vi "Dispose ListView.vi"(8 "error in (no error)":errorcluster caption="错误输入（无错误）", 11 "ListViewClass 输入":refnum<class "ListViewClass.lvclass"> caption="DNL_LabVIEW Object in") -> (0 "error out":errorcluster caption="错误输出", 3 "ListViewClass 输出":refnum<class "ListViewClass.lvclass"> caption="DNL_LabVIEW Object out")   [LabVIEW 2012, in "ListViewClass.lvclass"]
uses:
  ListViewClass.lvclass
  ListViewClass.lvclass/ListViewClass.ctl
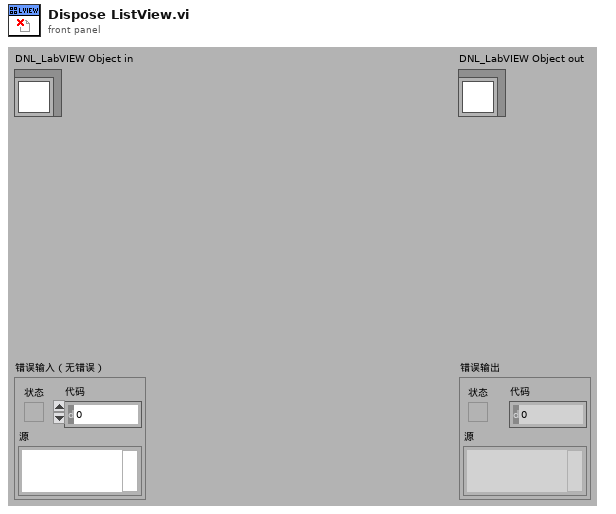
[diagram p1: front panel]
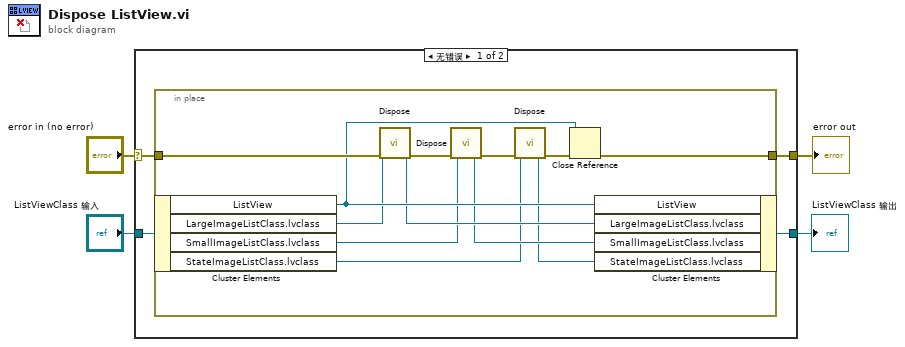
[diagram p0: block diagram]
diagram:
  n1 = case shown="无错误" "error in (no error)" {
    selector: "error in (no error)" -> [w8 w22]
    tunnel: [w7 w22] -> w3
    tunnel: [w5 w21] -> w1
    tunnel: "ListViewClass 输入" -> [w6 w21]
    frame No Error {
      n2 = in-place {
        in-place-border: w8 -> [w20]
        in-place-border: [w16] -> w7
        n3 = in-place-cluster #1(w6) -> ("ListView"=w15:refnum<k24>, "LargeImageListClass.lvclass"=w14:refnum<class "ImageListClass.lvclass">, "SmallImageListClass.lvclass"=w12:refnum<class "ImageListClass.lvclass">, "StateImageListClass.lvclass"=w10:refnum<class "ImageListClass.lvclass">)
        n4 = call "Dispose.vi"("error in (no error)"=w20, "ImageListClass 输入"=w14) -> ("error out"=w19:errorcluster, "ImageListClass 输出"=w13:refnum<class "ImageListClass.lvclass">)  [unwired: 8 in]
        n5 = call "Dispose.vi"("error in (no error)"=w19, "ImageListClass 输入"=w12) -> ("error out"=w18:errorcluster, "ImageListClass 输出"=w11:refnum<class "ImageListClass.lvclass">)  [unwired: 8 in]
        n6 = call "Dispose.vi"("error in (no error)"=w18, "ImageListClass 输入"=w10) -> ("error out"=w17:errorcluster, "ImageListClass 输出"=w9:refnum<class "ImageListClass.lvclass">)  [unwired: 8 in]
        n7 = Close Reference(reference=w15, error in (no error)=w17) -> (error out=w16:errorcluster)
        n8 = in-place-cluster #1("ListView"=w15, "LargeImageListClass.lvclass"=w13, "SmallImageListClass.lvclass"=w11, "StateImageListClass.lvclass"=w9) -> (w5:refnum<class "ListViewClass.lvclass">)
      }
    }
    frame Error {
    }
  }
  "error out" <- w3
  "ListViewClass 输出" <- w1
